vi "Xor.vi"(4 "b":bool, 5 "a":bool) -> (1 "out":bool)   [LabVIEW 2014]
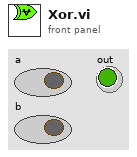
[diagram p1: front panel]
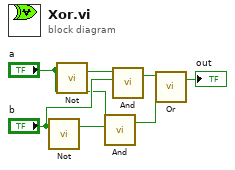
[diagram p0: block diagram]
diagram:
  n1 = call "Not.vi"("in"="b") -> ("out"=w5:bool)  [unwired: 2 in]
  n2 = call "Not.vi"("in"="a") -> ("out"=w7:bool)  [unwired: 2 in]
  n3 = call "And.vi"("b"=w5, "a"="a") -> ("out"=w3:bool)  [unwired: 3 in]
  n4 = call "And.vi"("b"="b", "a"=w7) -> ("out"=w4:bool)  [unwired: 3 in]
  n5 = call "Or.vi"("b"=w3, "a"=w4) -> ("out"=→"out":bool)  [unwired: 3 in]
